vi "OGB Replace Keywords in String.vi"(8 "error in (no error)":errorcluster, 9 "Value":string[](array[string]), 10 "Keyword":string[](array[string]), 11 "String in":string) -> (0 "error out":errorcluster, 3 "String out":string)   [LabVIEW 2011]
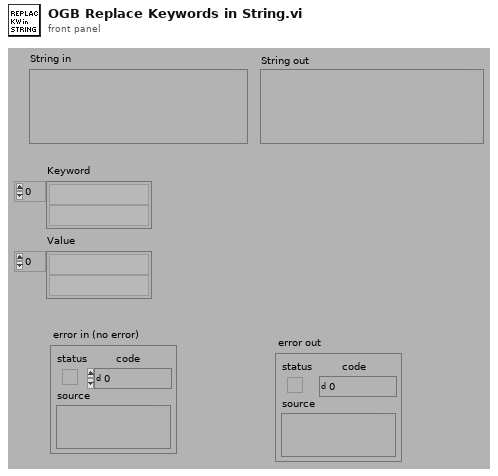
[diagram p1: front panel]
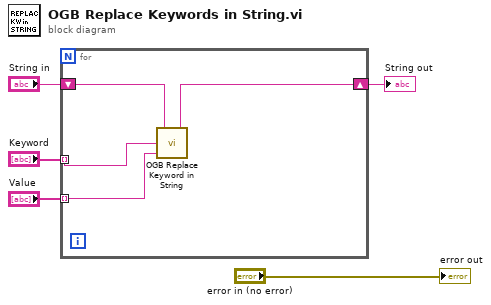
[diagram p0: block diagram]
diagram:
  n1 = for {
    tunnel: "Value" -> [w9] mode=indexing
    tunnel: "Keyword" -> [w8] mode=indexing
    shift-right: [w6] -> w4
    shift-left: "String in" -> [w7]
    n2 = call "OGB Replace Keyword in String.vi"("Value"=w9, "Keyword"=w8, "String"=w7) -> ("String out"=w6:string)
  }
  "String out" <- w4
  "error out" <- "error in (no error)"
